vi "Sub_Online_FEA_Delete_Pin_Location.vi"(10 "Pre-Pin Matrix":dbl[][](array[numeric]), 11 "Pin Location":i32) -> (3 "Post-Pin Matrix":dbl[][](array[numeric]))   [LabVIEW 2021]
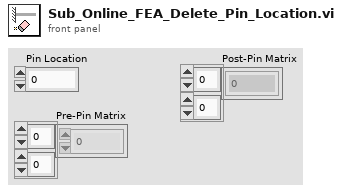
[diagram p1: front panel]
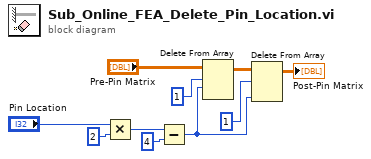
[diagram p0: block diagram]
diagram:
  n1 = Multiply(x="Pin Location", y=2) -> (x*y=w7:i32)
  n2 = Subtract(x=w7, y=4) -> (x-y=w1:i32)
  n3 = Delete From Array(array="Pre-Pin Matrix", length=1, index (row)=w1) -> (array with subset deleted=w4:dbl[][])  [unwired: 1 in, 1 out]
  n4 = Delete From Array(array=w4, length=1, index (col)=w1) -> (array with subset deleted=→"Post-Pin Matrix":dbl[][])  [unwired: 1 in, 1 out]
